vi "WriteVirtualStaveToFile.vi"() -> ()   [LabVIEW 2016]
uses:
  Controls/All_Enums/Enum_TypeDef_TapeType.ctl
  Controls/All_Enums/Enum_TypeDef_FidMarkers.ctl
  Controls/All_Enums/Enum_TypeDef_Sensors.ctl
  <vilib>/Utility/file.llb/Write Delimited Spreadsheet (DBL).vi
panel:
  out "Module fiducials in the XYZ stage's basis":T1(graph)=[{"Generated List of Module Coordinates"=[], "Generated List of Module Coordinates"=[]}, {"Generated List of Module Coordinates"=[-299.2110287057527, -202.7315011933668, -202.42767808647434, -298.9072055988603, -201.21150863720152, -104.73198112481558, -104.42815801792312, -200.90768553030907, -103.2119885686503, -6.732461056264299, -6.4286379493718755, -102.90816546175785, -5.212468500099078, 91.2670590122869, 91.57088211917932, -4.908645393206655, 92.78705156845217, 189.26657908083814, 189.57040218773056, 93.0908746753446, 190.7865716370033, 287.2660991493893, 287.5699222562817, 191.09039474389573, 288.7860917055545, 385.26561921794047, 385.5694423248329, 289.0899148124469, 386.7856117741057, 483.26513928649166, 483.5689623933841, 387.0894348809981, 484.7851318426569, 581.2646593550428, 581.5684824619352, 485.0889549495493, 582.7846519112081, 679.264179423594, 679.5680025304864, 583.0884750181006, 680.7841719797593, 777.2636994921454, 777.5675225990378, 681.0879950866517, 778.7836920483107, 875.2632195606966, 875.567042667589, 779.0875151552032, 876.7832121168619, 973.2627396292478, 973.5665627361402, 877.0870352237544], "Generated List of Module Coordinates"=[18.614201133837582, 18.312255796456228, 115.39178037048637, 115.69372570786773, 18.307498780361485, 18.00555344298013, 115.08507801701028, 115.38702335439163, 18.0007964268854, 17.698851089504046, 114.77837566353418, 115.08032100091555, 17.694094073409303, 17.39214873602795, 114.4716733100581, 114.77361864743946, 17.38739171993322, 17.08544638255185, 114.16497095658201, 114.46691629396337, 17.080689366457122, 16.778744029075767, 113.85826860310591, 114.16021394048727, 16.77398701298104, 16.47204167559967, 113.55156624962981, 113.85351158701118, 16.46728465950494, 16.165339322123586, 113.24486389615373, 113.54680923353509, 16.160582306028857, 15.858636968647488, 112.93816154267763, 113.240106880059, 15.85387995255276, 15.551934615171405, 112.63145918920155, 112.9334045265829, 15.547177599076676, 15.245232261695307, 112.32475683572545, 112.62670217310682, 15.240475245600578, 14.938529908219223, 112.01805448224937, 112.31999981963072, 14.933772892124495, 14.631827554743126, 111.71135212877327, 112.01329746615463]}, {"Generated List of Module Coordinates"=[-250.8193533961135, -152.81983332756232, -54.82031325901109, 43.17920680954012, 141.17872687809137, 239.1782469466425, 337.1777670151937, 435.1772870837449, 533.1768071522961, 631.1763272208473, 729.1758472893986, 827.1753673579499, 925.1748874265011], "Generated List of Module Coordinates"=[67.00299075216198, 66.69628839868588, 66.3895860452098, 66.0828836917337, 65.77618133825762, 65.46947898478152, 65.16277663130543, 64.85607427782934, 64.54937192435324, 64.24266957087715, 63.935967217401064, 63.62926486392497, 63.32256251044888]}]
  in  "Write?":bool
  in  "Stereo Angle [mrad]":dbl format="%#_13g"
  in  "N Modules":i32=13
  in  "Sensor Pattern":T2=enum."ATLAS12"
  in  "Module fiducial marker":T3=enum."Kapton Spacers"
  in  "Tape Type":T4=enum."Axial (Sutcliffe NP49-01-100 01-Mar-16)"
  # "WRITE VIRTUAL STAVE TO FILE Brandeis University - Brookhaven National Laboratory * ATLAS Phase II Inner Tracker Upgrade\nPrimary Author: Hannah Herde (hherde@brandeis.edu)"
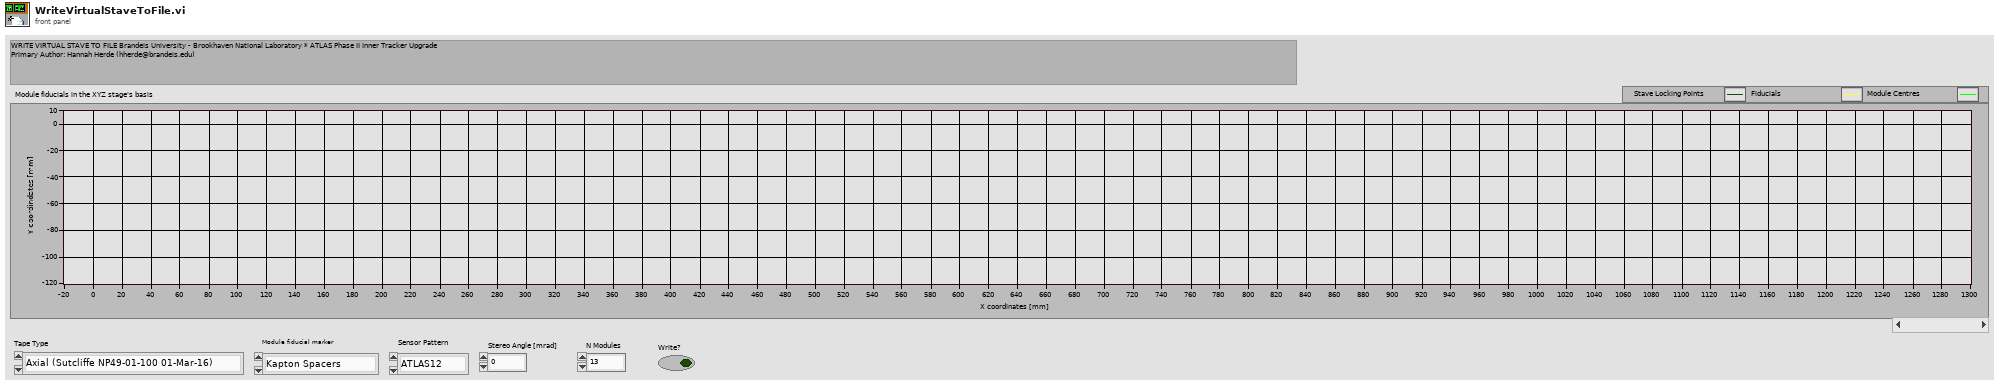
[diagram p1: front panel]
types:
  T1 = cluster{"Generated List of Module Coordinates":dbl[], "Generated List of Module Coordinates":dbl[]}[]
  T2 = typedef "Enum_TypeDef_Sensors.ctl" = enum16{"ATLAS07", "ATLAS12", "ATLAS12Slim", "ATLAS17LS"}
  T3 = typedef "Enum_TypeDef_FidMarkers.ctl" = enum16{"Mark B", "Mark C", "Bias Ring Corner", "Mark I (Slim/17)", "Mark E (Slim/17)", "Mark F (Slim/17)", "Mark G (Slim/17)", "Mark A (12)", "Kapton Spacers"}
  T4 = typedef "Enum_TypeDef_TapeType.ctl" = enum16{"Right stereo", "Left stereo", "Stereo (Sutcliffe NP49-01-100 01-Mar-16)", "Axial (Sutcliffe NP49-01-100 01-Mar-16)"}
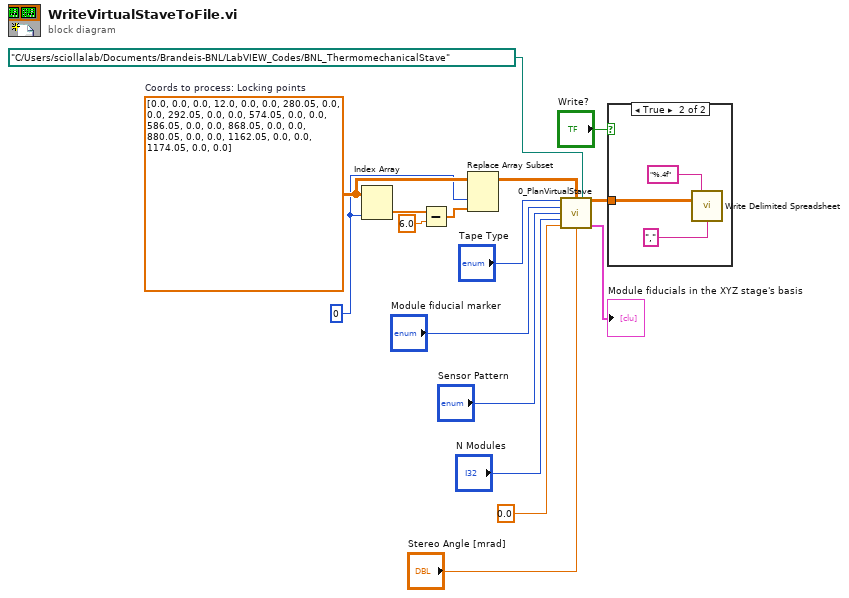
[diagram p0: block diagram]
diagram:
  w3 = 0 ("index")
  w4 = dbl[][] [[0.0, 0.0, 0.0], [12.0, 0.0, 0.0], [280.05, 0.0, 0.0], [292.05, 0.0, 0.0], [574.05, 0.0, 0.0], [586.05, 0.0, 0.0], [868.05, 0.0, 0.0], [880.05, 0.0, 0.0], [1162.05, 0.0, 0.0], [1174.05, 0.0, 0.0]]  # Coords to process: Locking points
  n1 = Index Array(array=w4, index (col)=w3) -> (element=w5:dbl[])  [unwired: 1 in]
  n2 = Subtract(x=w5, y=6.0) -> (x-y=w2:dbl[])
  n3 = Replace Array Subset(array=w4, new element=w2, index (col)=w3) -> (w1:dbl[][])  [unwired: 1 in]
  n4 = call "0_PlanVirtualStave.vi"("Tape Type"="Tape Type", "Stave Locking Points [mm]"=w1, "Code path"=path "C:/Users/sciollalab/Documents/Brandeis-BNL/LabVIEW_Codes/BNL_ThermomechanicalStave", "Module fiducial marker"="Module fiducial marker", "Sensor Pattern"="Sensor Pattern", "N Modules"="N Modules", "Working height [mm]"=0.0, "Stereo Angle [mrad]"="Stereo Angle [mrad]") -> ("Stave Basis: Coordinates of Fiducials on Modules"=w10:dbl[][], "Module fiducials in the Stave's basis"=→"Module fiducials in the XYZ stage's basis":T1)  [unwired: 5 in, 1 out]
  n5 = case shown="True" "Write?" {
    tunnel: w10 -> [_ w19]
    frame False {
    }
    frame True {
      n6 = call-poly <vilib>:"Write Delimited Spreadsheet.vi"("format (%.3f)"="%.4f", "2D data"=w19, "delimiter (\\t)"="," ("delimiter (\\t)")) -> ()  [unwired: 11 in, 2 out]
    }
  }
